vi "niFPGA Decimation.vi"(7 "reset":bool, 10 "dataRDYIn":bool, 11 "datain":fxp<+/-,16,16>) -> (0 "idle?":bool, 2 "dataReadyOut":bool, 3 "output data":fxp<+/-,18,1> format="%.18g")   [LabVIEW 2017]
uses:
  <vilib>/rvi/Emulation/niFpgaSctlEmulationGetInTimedLoop.vi
  <vilib>/Utility/error.llb/Clear Errors.vi
  <vilib>/rvi/Emulation/niFpgaSctlEmulationResourceMgr.vi
  <vilib>/rvi/Memory/Memory_Emulation/nirvimemoryEmulationManagerCache_SetValue.vi
  <vilib>/rvi/Emulation/niFpgaEmulationIsFPGAContextNoSignature.vi
  <vilib>/rvi/Memory/Memory_Emulation/nirvimemoryEmulationManagerCache_GetValue.vi
  <vilib>/rvi/Memory/Memory_Emulation/nirvimemoryEmulationManagerCache_ReleaseExclusive.vi
  <vilib>/rvi/Memory/Memory_Emulation/nirvimemoryEmulationManagerCache_InsertValue.vi
  <vilib>/rvi/Memory/Memory_Emulation/niFpgaMemoryEmulationValidateCache.vi
  <vilib>/rvi/Memory/Memory_Emulation/nirvimemoryEmulationManagerCache_MakeExclusive.vi
  <vilib>/rvi/Memory/Memory_Emulation/niFpgaMemoryEmulationCacheClearOnFirstRun.vi
  <vilib>/rvi/DataTransferAndStorage/Container/Common/niFpgaContainerGetUniqueNameForEmu.vi
  <vilib>/rvi/Emulation/niFpgaProcessEmulError.vi
  <vilib>/rvi/errors/nirviReportUnexpectedCaseInternalError (U32).vi
  <vilib>/rvi/DataTransferAndStorage/Container/Common/niFpgaContainerExecOnDevCompGetState.vi
  <vilib>/rvi/eio/common/nirviEmuReportErrorAndStop.vi
  <vilib>/rvi/DataTransferAndStorage/Container/Common/niFpgaContainerSetEmuInfo.vi
  <vilib>/rvi/DataTransferAndStorage/Container/XNode/niFpgaContainer.xnode
  <vilib>/rvi/Memory/Memory_Emulation/niFpgaMemoryEmulationRefIn.vi
  <vilib>/rvi/FXPMathLib/FxpMul/XNode/nifxpmath_Multiplier.xnode
  <vilib>/rvi/LocalResourceManager/LocalResourceManager.xnode
  <vilib>/rvi/FXPMathLib/sim/FxpSim.dll
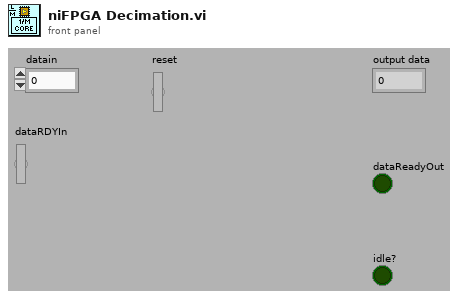
[diagram p1: front panel]
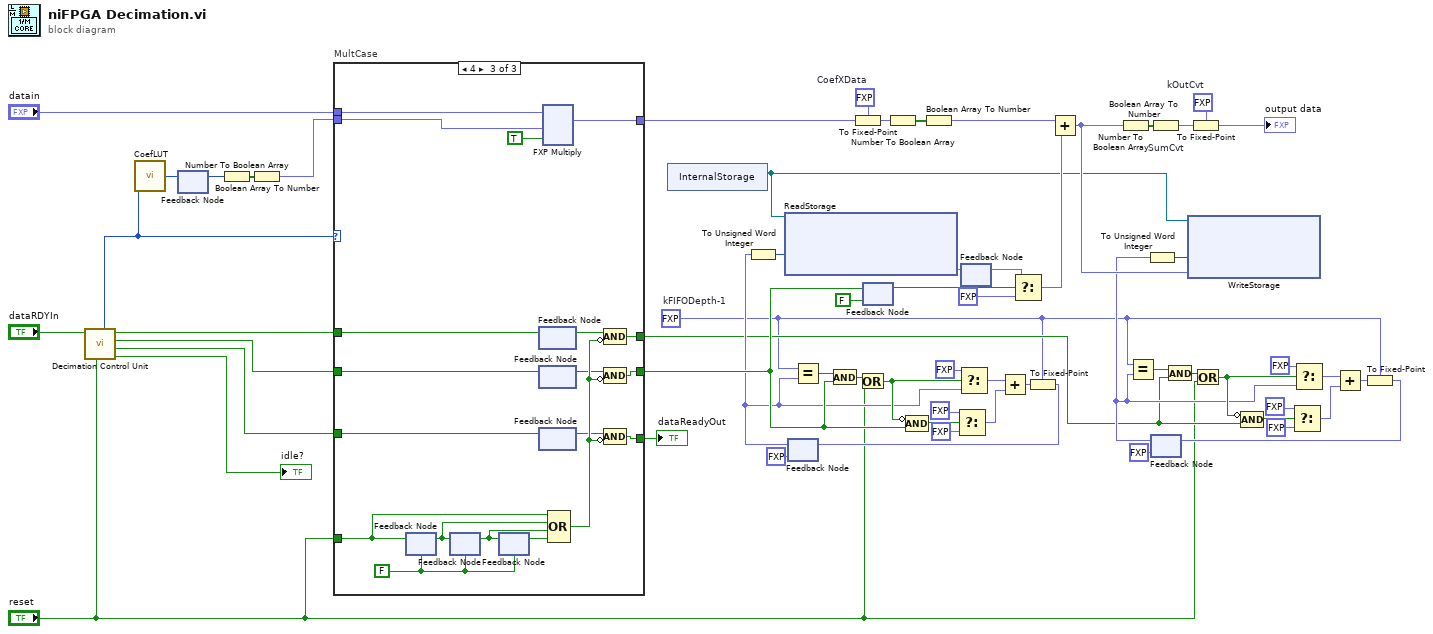
[diagram p0: block diagram]
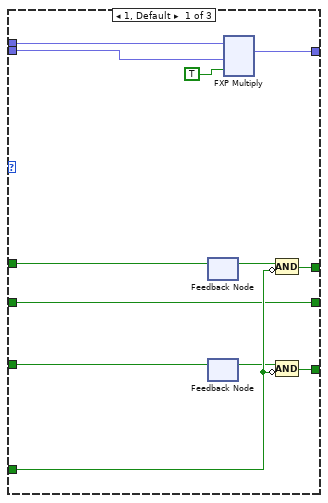
[diagram p2: hidden frame]
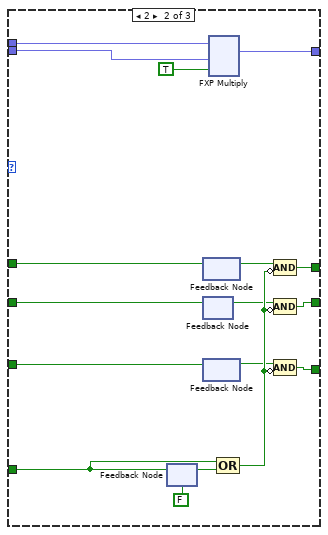
[diagram p3: hidden frame]
diagram:
  w39 = fxp<+/-,18,1> 0.0  # kOutCvt
  w54 = fxp<+/-,32,9> 0.0  # CoefXData
  w1 = fxp<+,5,5> 27.0  # kFIFODepth-1
  n1 = call "Decimation Control Unit"("reset"="reset", "dataRDYIn"="dataRDYIn") -> ("idle?"=→"idle?":bool, "dataReady?"=w45:bool, "read FIFO?"=w46:bool, "write FIFO?"=w47:bool, "coef idx"=w34:u16)  [unwired: 5 in]
  n2 = call "CoefLUT"("address"=w34) -> ("data out"=w32:i16)  [unwired: 8 in]
  n3 = feedback-in #1(w32) -> ()
  n4 = feedback #1() -> (w31:i16)  [unwired: 1 in]
  n5 = Number To Boolean Array(number=w31) -> (Boolean array=w36:bool[])
  n6 = Boolean Array To Number ("CoefCvt")(Boolean array=w36) -> (number=w35:fxp<+/-,16,1>)
  n7 = case "MultCase" shown="4" w34 {
    tunnel: "datain" -> [w72 w90 w109]
    tunnel: w35 -> [w71 w89 w108]
    tunnel: [w70 w88 w107] -> w50
    tunnel: w47 -> [w65 w80 w95]
    tunnel: [w68 w84 w100] -> w3
    tunnel: w46 -> [w66 w82 w92]
    tunnel: [w69 w86 w102] -> w49
    tunnel: w45 -> [w63 w78 w94]
    tunnel: [w66 w85 w101] -> w18
    tunnel: "reset" -> [w67 w76 w97]
    frame 1, Default {
      n8 = feedback #2() -> (w64:bool)  [unwired: 1 in]
      n9 = feedback-in #2(w65) -> ()
      n10 = feedback #3() -> (w62:bool)  [unwired: 1 in]
      n11 = feedback-in #3(w63) -> ()
      n12 = xnode ("FXP Multiply")("x"=w72, "y"=w71, "input valid"=TRUE) -> ("x*y"=w70:fxp<+/-,32,17>)  [unwired: 1 in, 2 out]
      n13 = Compound Arithmetic op=AND(w64, invert w67) -> (w68:bool)
      n14 = Compound Arithmetic op=AND(w62, invert w67) -> (w69:bool)
    }
    frame 2 {
      n15 = feedback-in #4(w76) -> ()
      n16 = feedback #4(FALSE ("reset")) -> (w74:bool)
      n17 = feedback #5() -> (w79:bool)  [unwired: 1 in]
      n18 = feedback-in #5(w80) -> ()
      n19 = feedback #6() -> (w81:bool)  [unwired: 1 in]
      n20 = feedback-in #6(w82) -> ()
      n21 = feedback #7() -> (w77:bool)  [unwired: 1 in]
      n22 = feedback-in #7(w78) -> ()
      n23 = xnode ("FXP Multiply")("x"=w90, "y"=w89, "input valid"=TRUE) -> ("x*y"=w88:fxp<+/-,32,17>)  [unwired: 1 in, 2 out]
      n24 = Compound Arithmetic op=OR(w76, w74) -> (w83:bool)
      n25 = Compound Arithmetic op=AND(w79, invert w83) -> (w84:bool)
      n26 = Compound Arithmetic op=AND(w81, invert w83) -> (w85:bool)
      n27 = Compound Arithmetic op=AND(w77, invert w83) -> (w86:bool)
    }
    frame 4 {
      w98 = FALSE ("reset")
      n28 = feedback-in #8(w97) -> ()
      n29 = feedback #8(w98) -> (w103:bool)
      n30 = feedback-in #9(w103) -> ()
      n31 = feedback #9(w98) -> (w104:bool)
      n32 = feedback-in #10(w104) -> ()
      n33 = feedback #10(w98) -> (w105:bool)
      n34 = feedback-in #11(w95) -> ()
      n35 = feedback #11() -> (w96:bool)  [unwired: 1 in]
      n36 = feedback #12() -> (w91:bool)  [unwired: 1 in]
      n37 = feedback-in #12(w92) -> ()
      n38 = feedback #13() -> (w93:bool)  [unwired: 1 in]
      n39 = feedback-in #13(w94) -> ()
      n40 = xnode ("FXP Multiply")("x"=w109, "y"=w108, "input valid"=TRUE) -> ("x*y"=w107:fxp<+/-,32,17>)  [unwired: 1 in, 2 out]
      n41 = Compound Arithmetic op=OR(w97, w103, w104, w105) -> (w99:bool)
      n42 = Compound Arithmetic op=AND(w96, invert w99) -> (w100:bool)
      n43 = Compound Arithmetic op=AND(w91, invert w99) -> (w101:bool)
      n44 = Compound Arithmetic op=AND(w93, invert w99) -> (w102:bool)
    }
  }
  "dataReadyOut" <- w49
  n45 = xnode "InternalStorage"() -> ("Memory Out"=w33:refnum<k21>)
  n46 = feedback #14(fxp<+,1,1> 0.0) -> (w17:fxp<+,5,5>)
  n47 = To Unsigned Word Integer(number=w17) -> (unsigned 16bit integer=w53:u16)
  n48 = xnode "ReadStorage"("Address"=w53, "Memory In"=w33) -> ("Data"=w61:fxp<+/-,32,32>)  [unwired: 1 out]
  n49 = Equal?(x=w1, y=w17) -> (x = y?=w29:bool)
  n50 = And(x=w29, y=w18) -> (x .and. y?=w28:bool)
  n51 = To Fixed-Point(fixed-point type=w54, number=w50) -> (fixed-point=w56:fxp<+/-,32,9>)
  n52 = Or(x=w28, y="reset") -> (x .or. y?=w27:bool)
  n53 = feedback-in #15(w18) -> ()
  n54 = feedback #15(FALSE ("read FIFO?")) -> (w52:bool)
  n55 = Number To Boolean Array(number=w56) -> (Boolean array=w57:bool[])
  n56 = Compound Arithmetic op=AND(invert w27, w18) -> (w24:bool)
  n57 = Boolean Array To Number(Boolean array=w57) -> (number=w55:fxp<+/-,32,32>)
  n58 = Select(t=fxp<+,1,1> 1.0 ("y"), s=w24, f=fxp<+,1,1> 0.0) -> (s? t:f=w21:fxp<+,1,1>)
  n59 = Select(t=fxp<+,1,1> 0.0 ("y"), s=w27, f=w17) -> (s? t:f=w25:fxp<+,5,5>)
  n60 = feedback-in #16(w61) -> ()
  n61 = feedback #16() -> (w58:fxp<+/-,32,32>)  [unwired: 1 out]
  n62 = Add(x=w25, y=w21) -> (x+y=w20:fxp<+,6,6>)
  n63 = Select(t=w58, s=w52, f=fxp<+/-,32,32> 0.0) -> (s? t:f=w59:fxp<+/-,32,32>)
  n64 = To Fixed-Point(fixed-point type=w1, number=w20) -> (fixed-point=w19:fxp<+,5,5>)
  n65 = feedback-in #14(w19) -> ()
  n66 = Add(x=w55, y=w59) -> (x+y=w38:fxp<+/-,32,32>)
  n67 = Number To Boolean Array(number=w38) -> (Boolean array=w41:bool[])
  n68 = Boolean Array To Number "SumCvt"(Boolean array=w41) -> (number=w40:fxp<+/-,32,17>)
  n69 = feedback #17(fxp<+,1,1> 0.0) -> (w4:fxp<+,5,5>)
  n70 = Equal?(x=w1, y=w4) -> (x = y?=w6:bool)
  n71 = To Unsigned Word Integer(number=w4) -> (unsigned 16bit integer=w48:u16)
  n72 = And(x=w6, y=w3) -> (x .and. y?=w7:bool)
  n73 = xnode "WriteStorage"("Address"=w48, "Data"=w38, "Memory In"=w33) -> ()  [unwired: 1 out]
  n74 = To Fixed-Point(fixed-point type=w39, number=w40) -> (fixed-point=→"output data":fxp<+/-,18,1>)
  n75 = Or(x=w7, y="reset") -> (x .or. y?=w8:bool)
  n76 = Compound Arithmetic op=AND(invert w8, w3) -> (w11:bool)
  n77 = Select(t=fxp<+,1,1> 1.0 ("y"), s=w11, f=fxp<+,1,1> 0.0) -> (s? t:f=w14:fxp<+,1,1>)
  n78 = Select(t=fxp<+,1,1> 0.0 ("y"), s=w8, f=w4) -> (s? t:f=w10:fxp<+,5,5>)
  n79 = Add(x=w10, y=w14) -> (x+y=w15:fxp<+,6,6>)
  n80 = To Fixed-Point(fixed-point type=w1, number=w15) -> (fixed-point=w16:fxp<+,5,5>)
  n81 = feedback-in #17(w16) -> ()
